vi "Transceiver Thread.Set Thread Parameters.vi"(10 "Thread Parameters":refnum<class "Thread Parameters.lvclass">, 11 "Transceiver Thread in":refnum<class "Transceiver Thread.lvclass">) -> (3 "Transceiver Thread out":refnum<class "Transceiver Thread.lvclass">)   [LabVIEW 2017, in "DSF.Engine.lvlib" / "Transceiver Thread.lvclass"]
uses:
  Transceiver Thread.lvclass
  Thread Parameters/Thread Parameters.lvclass
  Transceiver Thread.lvclass/Transceiver Thread.ctl
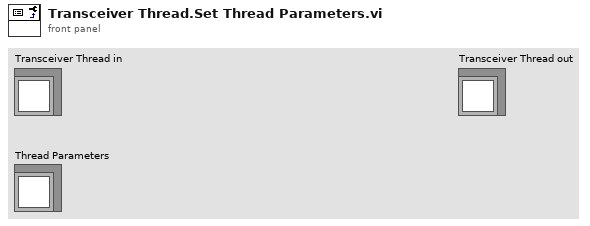
[diagram p1: front panel]
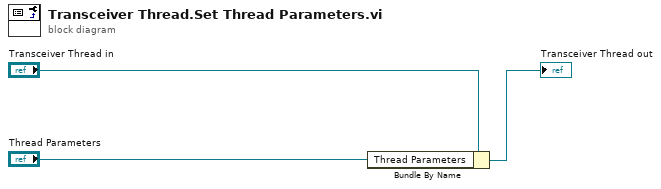
[diagram p0: block diagram]
diagram:
  n1 = Bundle By Name(cluster="Transceiver Thread in", "Thread Parameters"="Thread Parameters") -> (→"Transceiver Thread out":refnum<class "Transceiver Thread.lvclass">)
